vi "Func1.vi"(8 "x":dbl, 11 "y":dbl) -> (3 "result":dbl)   [LabVIEW 2014, in "Plugin1.lvlib"]
uses:
  Plugin1.lvlib
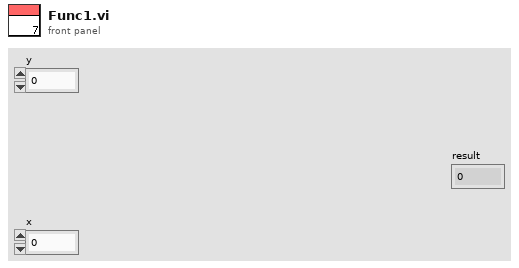
[diagram p1: front panel]
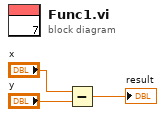
[diagram p0: block diagram]
diagram:
  n1 = Subtract(x="x", y="y") -> (x-y=→"result":dbl)
